vi "EXO1.vi"() -> ()   [LabVIEW 2020]
panel:
  in  "Nr of Analog Inputs":i16=2
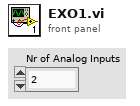
[diagram p1: front panel]
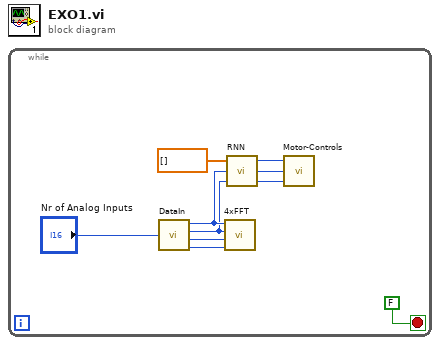
[diagram p0: block diagram]
diagram:
  n1 = while {
    stop <- FALSE stop-if-true
    n2 = call "DataIn.vi"("Nr of Analog Inputs"="Nr of Analog Inputs") -> ("AnalogIn0"=w6:u16, "AnalogIn1"=w5:u16, "AnalogIn2"=w9:u16, "AnalogIn3"=w8:u16)
    n3 = call "4xFFT.vi"("Input 4"=w8, "Input 3"=w9, "Input 2"=w5, "Input 1"=w6) -> ()  [unwired: 4 in, 4 out]
    n4 = call "RNN.vi"("Input 2"=w5, "Input 1"=w6, "Weights"=sgl[] []) -> ("Downwards"=w2:u16, "Still"=w3:u16, "Upwards"=w4:u16)
    n5 = call "Motor-Controls.vi"("Downwards"=w2, "Still"=w3, "Upwards"=w4) -> ()  [unwired: 6 in]
  }
